vi "Energy Detection.vi"() -> ()   [LabVIEW 2012]
uses:
  <vilib>/measure/maspectr.llb/FFT Power Spectrum and PSD for 1 Chan.vi
  <instrlib>/niUSRP/niUSRP Fetch Rx Data (CDB Cluster).vi
  <vilib>/addons/Modulation/Digital/General/MT Generate PSK System Parameters(M).vi
  <instrlib>/niUSRP/niUSRP Write Tx Data (CDB Cluster).vi
  <vilib>/addons/Modulation/niDMT.lvlib
  <vilib>/measure/NI_MAPro.lvlib
panel:
  out "Power Spectrum / PSD":cluster{"f0":dbl, "df":dbl, "magnitude":dbl[]} {"magnitude" format="%.2p"; "f0" format="%0.2p"; "df" format="%0.2p"}
  out "SNR":dbl
  out "x/y":dbl
  in  "IQ rate 2":dbl=100000.0 format="%#_6p"
  in  "gain":dbl format="%#_6f"
  out "x+y 2":dbl
  out "CH1 is Free":bool
  out "CH2 is Free":bool
  out "CH3 is Free":bool
  out "CH4 is Free":bool
  out "String":string
  in  "millisecond multiple":u32
  out "millisecond timer value":u32
  out "Message Text 2":string
  out "Symbol Rate\n[symbols/sec]":dbl=25000.0 format="%#.6p"
  in  "BPSK System Parameters 9":T1={"Samples per Symbol"=8, "symbol map"=[], "Differential PSK"=enum."disable", "PSK type"=0} caption="BPSK System Parameters" {"PSK type" items=["normal", "shifted", "offset"]; "symbol map" format="%.3f"}
  in  "BPSK System Parameters 8":T1={"Samples per Symbol"=8, "symbol map"=[], "Differential PSK"=enum."disable", "PSK type"=0} caption="BPSK System Parameters" {"PSK type" items=["normal", "shifted", "offset"]; "symbol map" format="%.3f"}
  in  "BPSK System Parameters 7":T1={"Samples per Symbol"=8, "symbol map"=[], "Differential PSK"=enum."disable", "PSK type"=0} caption="BPSK System Parameters" {"PSK type" items=["normal", "shifted", "offset"]; "symbol map" format="%.3f"}
  in  "BPSK System Parameters 6":T1={"Samples per Symbol"=8, "symbol map"=[], "Differential PSK"=enum."disable", "PSK type"=0} caption="BPSK System Parameters" {"PSK type" items=["normal", "shifted", "offset"]; "symbol map" format="%.3f"}
  in  "BPSK System Parameters 5":T1={"Samples per Symbol"=8, "symbol map"=[], "Differential PSK"=enum."disable", "PSK type"=0} caption="BPSK System Parameters" {"PSK type" items=["normal", "shifted", "offset"]; "symbol map" format="%.3f"}
  in  "BPSK System Parameters 4":T1={"Samples per Symbol"=8, "symbol map"=[], "Differential PSK"=enum."disable", "PSK type"=0} caption="BPSK System Parameters" {"PSK type" items=["normal", "shifted", "offset"]; "symbol map" format="%.3f"}
  in  "BPSK System Parameters 3":T1={"Samples per Symbol"=8, "symbol map"=[], "Differential PSK"=enum."disable", "PSK type"=0} caption="BPSK System Parameters" {"PSK type" items=["normal", "shifted", "offset"]; "symbol map" format="%.3f"}
  in  "Tab Control":T2(tab)
  in  "Enter control signal (1,2 or 3)":string
  in  "Packet Parameters":T3={"Guard Bits "=30, "Sync Bits"=20, "Message Bits"=128}
  in  "Packet Pad \n[samples]":i32=200
  in  "Blank Frame \n[samples]":i32=500
  out "Number of Packets in Message":i32=46
  in  "PN sequence order\nfor Sync Bits":i32=31 caption="PN sequence order (9)"
  in  "Packet Repeat":i32=2
  in  "Pulse Shaping Filter Parameters":T4={"Alpha"=0.5, "Filter Length"=6, "TX Filter"=enum."Root Raised Cos"} caption="Pulse Shaping Filter" {"Alpha" format="%.2f"}
  in  "USRP IP address":refnum<k15>="192.168.10.2"
  out "error out":errorcluster
  in  "Queue Length":i32=10
  in  "stop":bool
  out "result":bool
  out "Constellation Graph":T5(graph)
  in  "autoscale":bool
  in  "millisecond multiple 2":u32
  out "millisecond timer value 2":u32
  out "x = y?":bool
  out "Boolean":bool
  out "M-PSK (4)":i32
  out "Enter control signal (1,2 or 3) 2":string
  out "Tx Frequency [Hz]":dbl
  out "x+y":dbl
  in  "Carrier Frequency":dbl
  in  "active antenna":string
  in  "IQ rate":dbl=100000.0 format="%#_6p"
  out "coerced carrier frequency":dbl=100000.0 format="%#_6p"
  out "coerced gain":dbl format="%#_6f"
  # "Guard\nBand"
  # "Sync\nSeq"
  # "Packet\nNumber"
  # "Pad\nData"
  # "Blank\nFrame"
  # "Data"
types:
  T1 = cluster{"Samples per Symbol":i32, "symbol map":cdb[], "Differential PSK":enum16{"disable", "enable"}, "PSK type":u16}
  T2 = enum32{"Specify Message", "Specify Packet", "Specify Modulation", "Tx Parameters", "Debug"}
  T3 = cluster{"Guard Bits ":i32, "Sync Bits":i32, "Message Bits":i32}
  T4 = cluster{"Alpha":dbl, "Filter Length":i32, "TX Filter":enum16{"none", "Raised Cosine", "Root Raised Cos", "Gaussian"}}
  T5 = cluster{"Decimated Array":dbl[], "Decimated Array":dbl[]}[]
  T6 = cluster{"samples per symbol (16)":i32, "symbol map":cdb[], "differential PSK":enum16{"disable", "enable"}, "PSK type":u16}
  T7 = cluster{"s? t:f":cluster{"t0":dbl, "dt":dbl, "Y":cdb[]}, i32}
  T8 = cluster{"output complex waveform":cluster{"t0":dbl, "dt":dbl, "Y":cdb[]}, i32}
  T9 = cluster{"constellation":dbl[], "oversampled data":dbl[]}[]
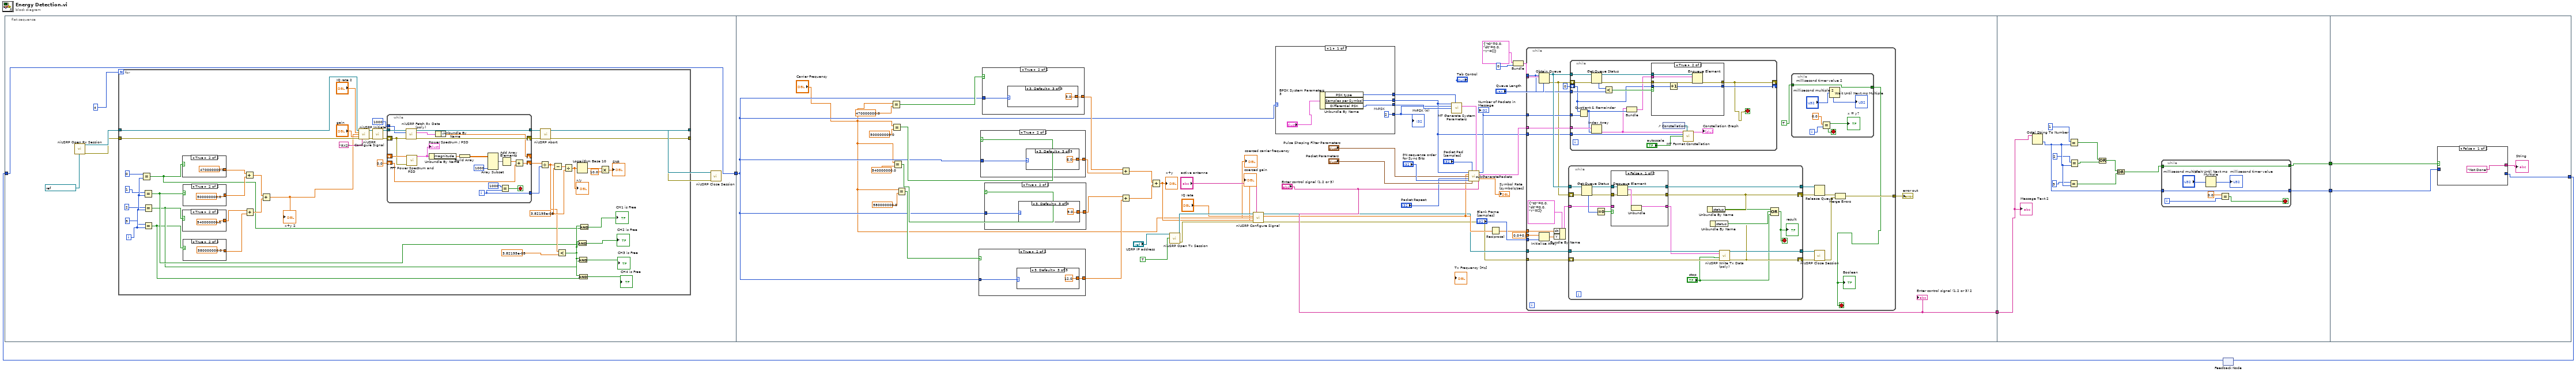
[diagram p0: block diagram]
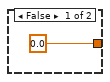
[diagram p2: hidden frame]
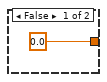
[diagram p3: hidden frame]
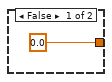
[diagram p4: hidden frame]
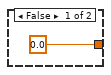
[diagram p5: hidden frame]
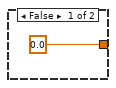
[diagram p6: hidden frame]
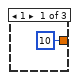
[diagram p7: hidden frame]
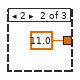
[diagram p8: hidden frame]
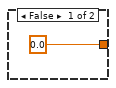
[diagram p9: hidden frame]
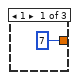
[diagram p10: hidden frame]
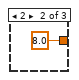
[diagram p11: hidden frame]
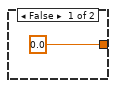
[diagram p12: hidden frame]
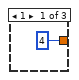
[diagram p13: hidden frame]
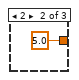
[diagram p14: hidden frame]
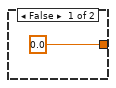
[diagram p15: hidden frame]
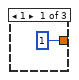
[diagram p16: hidden frame]
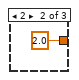
[diagram p17: hidden frame]
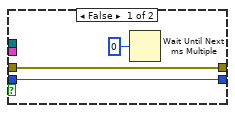
[diagram p18: hidden frame]
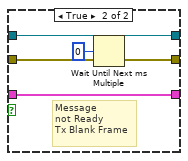
[diagram p19: hidden frame]
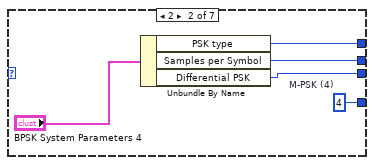
[diagram p20: hidden frame]
diagram:
  n1 = flat-sequence {
    tunnel: w1 -> [w13]
    tunnel: [w13] -> w2
    tunnel: ["Enter control signal (1,2 or 3)"] -> w6
    tunnel: w2 -> [w94]
    tunnel: w6 -> [w283]
    tunnel: [w285] -> w5
    tunnel: [w284] -> w4
    tunnel: w5 -> [w304]
    tunnel: w4 -> [w303]
    tunnel: [w302] -> w3
    frame #0 {
      n2 = call <instrlib>:"niUSRP Open Rx Session.vi"("device names"=refnum<k15> "192.168.10.4") -> ("session handle out"=w12:refnum<k15>, "error out"=w11:errorcluster)  [unwired: 13 in]
      n3 = for {
        N: 4 -> [_]
        tunnel: w12 -> [w59]
        tunnel: w11 -> [w56]
        tunnel: [w42] -> w8
        tunnel: [w41] -> w7
        i -> [w36]
        w38 = 3.82195e-05 ("y")
        n4 = Equal?(x=0, y=w36) -> (x = y?=w21:bool)
        n5 = Equal?(x=1, y=w36) -> (x = y?=w20:bool)
        n6 = Equal?(x=2, y=w36) -> (x = y?=w19:bool)
        n7 = Equal?(x=3, y=w36) -> (x = y?=w18:bool)
        n8 = case shown="True" w21 {
          tunnel: [0.0 470000000.0] -> w31
          frame False {
          }
          frame True {
          }
        }
        n9 = case shown="True" w19 {
          tunnel: [0.0 540000000.0] -> w29
          frame False {
          }
          frame True {
          }
        }
        n10 = case shown="True" w20 {
          tunnel: [0.0 500000000.0] -> w30
          frame False {
          }
          frame True {
          }
        }
        n11 = case shown="True" w18 {
          tunnel: [0.0 580000000.0] -> w26
          frame False {
          }
          frame True {
          }
        }
        n12 = Add(x=w31, y=w30) -> (x+y=w28:dbl)
        n13 = Add(x=w29, y=w26) -> (x+y=w27:dbl)
        n14 = Add(x=w28, y=w27) -> (x+y=w23:dbl)
        "x+y 2" <- w23
        n15 = call <instrlib>:"niUSRP Configure Signal.vi"("session handle"=w59, "IQ rate"="IQ rate 2", "carrier frequency"=w23, "gain"="gain", "error in (no error)"=w56, "active antenna"="RX2") -> ("session handle out"=w58:refnum<k15>, "error out"=w57:errorcluster)  [unwired: 5 in, 3 out]
        n16 = call <instrlib>:"niUSRP Initiate.vi"("session handle"=w58, "error in (no error)"=w57) -> ("session handle out"=w55:refnum<k15>, "error out"=w54:errorcluster)  [unwired: 12 in]
        n17 = while {
          tunnel: w55 -> [w86]
          shift-right: [w70] -> w53
          shift-left: w54 -> [w83]
          tunnel: [w85] -> w52
          shift-right: [w68] -> _
          shift-left: _ -> [w84]
          shift-right: [w77] -> w50
          shift-left: 0.0 -> [w78]
          tunnel: [w72] -> w49
          tunnel: 1000 -> [w75]
          i -> [w72]
          stop <- w71 stop-if-true
          n18 = call-poly <instrlib>:"niUSRP Fetch Rx Data (poly).vi"("session handle"=w86, "number of samples"=w75, "error in (no error)"=w83) -> ("session handle out"=w85:refnum<k15>, "data"=w69:cluster{"t0":dbl, "dt":dbl, "Y":cdb[]}, "error out"=w70:errorcluster)  [unwired: 9 in, 1 out]
          n19 = call-poly <vilib>:"FFT Power Spectrum and PSD.vi"("error in (no error)"=w83, "time signal"=w84) -> ("Power Spectrum / PSD"=w82:cluster{"f0":dbl, "df":dbl, "magnitude":dbl[]})  [unwired: 6 in, 3 out]
          "Power Spectrum / PSD" <- w82
          n20 = Unbundle By Name(w82) -> ("magnitude"=w81:dbl[])
          n21 = Unbundle By Name(w69) -> ("Y"=w68:cdb[])
          n22 = Build Array(w81) -> (w80:dbl[][])
          n23 = Array Subset(array=w80, length (col)=1000 ("length")) -> (w79:dbl[][])  [unwired: 3 in]
          n24 = Equal?(x=1000, y=w72) -> (x = y?=w71:bool)
          n25 = Add Array Elements(numeric array=w79) -> (sum=w76:dbl)
          n26 = Add(x=w76, y=w78) -> (x+y=w77:dbl)
        }
        n27 = Divide(x=w50, y=w49) -> (x/y=w25:dbl)
        n28 = call <instrlib>:"niUSRP Abort.vi"("session handle"=w52, "error in (no error)"=w53) -> ("session handle out"=w42:refnum<k15>, "error out"=w41:errorcluster)  [unwired: 12 in]
        n29 = Subtract(x=w25, y=w38) -> (x-y=w37:dbl)
        n30 = Less?(x=w25, y=3.82195e-05) -> (x < y?=w22:bool)
        n31 = Divide(x=w37, y=w38) -> (x/y=w48:dbl)
        "x/y" <- w48
        n32 = Logarithm Base 10(1:w48) -> (0:w47:dbl)
        n33 = And(x=w22, y=w20) -> (x .and. y?=→"CH2 is Free":bool)
        n34 = And(x=w22, y=w19) -> (x .and. y?=→"CH3 is Free":bool)
        n35 = And(x=w22, y=w18) -> (x .and. y?=→"CH4 is Free":bool)
        n36 = And(x=w22, y=w21) -> (x .and. y?=→"CH1 is Free":bool)
        n37 = Multiply(x=w47, y=10.0) -> (x*y=→"SNR":dbl)
      }
      n38 = call <instrlib>:"niUSRP Close Session.vi"("session handle"=w8, "error in (no error)"=w7) -> ()  [unwired: 13 in, 1 out]
    }
    frame #1 {
      n39 = Equal?(x="Carrier Frequency", y=470000000.0) -> (x = y?=w95:bool)
      n40 = Equal?(x="Carrier Frequency", y=500000000.0) -> (x = y?=w96:bool)
      n41 = Equal?(x="Carrier Frequency", y=540000000.0) -> (x = y?=w97:bool)
      n42 = Equal?(x="Carrier Frequency", y=580000000.0) -> (x = y?=w98:bool)
      n43 = case shown="True" w98 {
        tunnel: [0.0 w138] -> w103
        tunnel: w94 -> [_ w139]
        frame False {
        }
        frame True {
          n44 = case shown="3, Default" w139 {
            tunnel: [10 11.0 12.0] -> w138
            frame 1 {
            }
            frame 2 {
            }
            frame 3, Default {
            }
          }
        }
      }
      n45 = case shown="True" w96 {
        tunnel: [0.0 w150] -> w105
        tunnel: w94 -> [_ w151]
        frame False {
        }
        frame True {
          n46 = case shown="3, Default" w151 {
            tunnel: [4 5.0 6.0] -> w150
            frame 1 {
            }
            frame 2 {
            }
            frame 3, Default {
            }
          }
        }
      }
      n47 = case shown="True" w95 {
        tunnel: [0.0 w156] -> w106
        tunnel: w94 -> [_ w157]
        frame False {
        }
        frame True {
          n48 = case shown="3, Default" w157 {
            tunnel: [1 2.0 3.0] -> w156
            frame 1 {
            }
            frame 2 {
            }
            frame 3, Default {
            }
          }
        }
      }
      n49 = case shown="True" w97 {
        tunnel: [0.0 w144] -> w104
        tunnel: w94 -> [_ w145]
        frame False {
        }
        frame True {
          n50 = case shown="3, Default" w145 {
            tunnel: [7 8.0 9.0] -> w144
            frame 1 {
            }
            frame 2 {
            }
            frame 3, Default {
            }
          }
        }
      }
      n51 = Add(x=w106, y=w105) -> (x+y=w108:dbl)
      n52 = Add(x=w104, y=w103) -> (x+y=w107:dbl)
      n53 = Add(x=w108, y=w107) -> (x+y=w93:dbl)
      "x+y" <- w93
      n54 = call <instrlib>:"niUSRP Open Tx Session.vi"("device names"="USRP IP address", "reset"=TRUE) -> ("session handle out"=w111:refnum<k15>, "error out"=w112:errorcluster)  [unwired: 12 in]
      n55 = call <instrlib>:"niUSRP Configure Signal.vi"("session handle"=w111, "IQ rate"="IQ rate", "carrier frequency"="Carrier Frequency", "gain"=w93, "error in (no error)"=w112, "active antenna"="active antenna") -> ("session handle out"=w110:refnum<k15>, "coerced IQ rate"=w113:dbl, "coerced carrier frequency"=→"coerced carrier frequency":dbl, "coerced gain"=→"coerced gain":dbl, "error out"=w109:errorcluster)  [unwired: 5 in]
      n56 = case shown="1" w94 {
        tunnel: [w249 w254 w261 w266 w271 w277 w280] -> w117
        tunnel: [w250 w255 w260 w265 w270 w276 w281] -> w136
        tunnel: [w252 w257 w262 w267 w269 w275 0 ("M-PSK (4)")] -> w128
        tunnel: [w251 w256 w259 w264 w272 w274 w282] -> w122
        frame 1 {
          w252 = 2  # M-PSK
          n57 = Unbundle By Name("BPSK System Parameters 3") -> ("PSK type"=w251:u16, "Samples per Symbol"=w249:i32, "Differential PSK"=w250:enum16{"disable", "enable"})
        }
        frame 2 {
          w257 = 4  # M-PSK (4)
          n58 = Unbundle By Name("BPSK System Parameters 4") -> ("PSK type"=w256:u16, "Samples per Symbol"=w254:i32, "Differential PSK"=w255:enum16{"disable", "enable"})
        }
        frame 4 {
          w262 = 4  # M-PSK (4)
          n59 = Unbundle By Name("BPSK System Parameters 5") -> ("PSK type"=w259:u16, "Samples per Symbol"=w261:i32, "Differential PSK"=w260:enum16{"disable", "enable"})
        }
        frame 5 {
          w267 = 4  # M-PSK (4)
          n60 = Unbundle By Name("BPSK System Parameters 6") -> ("PSK type"=w264:u16, "Samples per Symbol"=w266:i32, "Differential PSK"=w265:enum16{"disable", "enable"})
        }
        frame 3, Default {
          w269 = 8  # M-PSK (4)
          n61 = Unbundle By Name("BPSK System Parameters 7") -> ("PSK type"=w272:u16, "Samples per Symbol"=w271:i32, "Differential PSK"=w270:enum16{"disable", "enable"})
        }
        frame 6 {
          w275 = 16  # M-PSK (4)
          n62 = Unbundle By Name("BPSK System Parameters 8") -> ("PSK type"=w274:u16, "Samples per Symbol"=w277:i32, "Differential PSK"=w276:enum16{"disable", "enable"})
        }
        frame 7 {
          n63 = Unbundle By Name("BPSK System Parameters 9") -> ("PSK type"=w282:u16, "Samples per Symbol"=w280:i32, "Differential PSK"=w281:enum16{"disable", "enable"})
        }
      }
      "M-PSK (4)" <- w128
      n64 = call-poly <vilib>:"MT Generate System Parameters.vi"("samples per symbol (16)"=w117, "PSK type"=w122, "M-PSK (4)"=w128, "differential PSK"=w136) -> ("PSK system parameters"=w123:T6)  [unwired: 9 in, 2 out]
      n65 = call "subGeneratePackets.vi"("Samples per Symbol"=w117, "Packet Pad \n[samples]"="Packet Pad \n[samples]", "PSK system parameters"=w123, "Tx IQ Sampling\nRate [s/sec]"=w113, "Pulse Shaping Filter Parameters"="Pulse Shaping Filter Parameters", "Packet Repeat"="Packet Repeat", "PN sequence order\nfor Sync Bits"="PN sequence order\nfor Sync Bits", "Packet Parameters"="Packet Parameters", "Message Text"="Enter control signal (1,2 or 3)") -> ("Number of Packets"=w127:i32, "Packets"=w130:cluster{"t0":dbl, "dt":dbl, "Y":cdb[]}[], "Symbol Rate"=→"Symbol Rate\n[symbols/sec]":dbl)  [unwired: 4 in]
      "Number of Packets in Message" <- w127
      n66 = Reciprocal(x=w113) -> (1/x=w129:dbl)
      n67 = Bundle("s? t:f"=cluster{"t0":dbl, "dt":dbl, "Y":cdb[]} {"t0"=0.0, "dt"=0.0, "Y"=[]}, 0) -> (w132:T7)  [unwired: 1 in]
      n68 = while {
        tunnel: cdb 0.0+0.0i ("element") -> [w185]
        tunnel: "Blank Frame \n[samples]" -> [w184]
        tunnel: w132 -> [w178]
        tunnel: "Queue Length" -> [w176]
        tunnel: w130 -> [w175]
        tunnel: w109 -> [w174]
        tunnel: w129 -> [w171]
        tunnel: w110 -> [w170]
        tunnel: w127 -> [w169]
        tunnel: [w164] -> w121
        tunnel: w117 -> [w163]
        stop <- w161 stop-if-true
        n69 = Obtain Queue(max queue size (-1, unlimited)=w176, element data type=w178) -> (queue out=w183:refnum<queue>, error out=w167:errorcluster)  [unwired: 3 in, 1 out]
        n70 = Initialize Array(w185, w184) -> (w182:cdb[])
        n71 = Bundle By Name(cluster=cluster{"t0":dbl, "dt":dbl, "Y":cdb[]} {"t0"=0.0, "dt"=0.0, "Y"=[]} ("s? t:f"), "dt"=w171, "Y"=w182) -> (w181:cluster{"t0":dbl, "dt":dbl, "Y":cdb[]})
        n72 = while {
          tunnel: w170 -> [w228]
          shift-right: [w225] -> w173
          shift-left: w174 -> [w229]
          tunnel: w183 -> [w237]
          tunnel: w181 -> [w234]
          tunnel: [w233] -> w180
          tunnel: [w227] -> w172
          shift-right: [w223] -> w179
          shift-left: w167 -> [w230]
          stop <- w220 stop-if-true
          n73 = Get Queue Status(queue=w237, error in (no error)=w230) -> (queue out=w232:refnum<queue>, error out=w231:errorcluster, # elements in queue=w236:i32)  [unwired: 1 in, 5 out]
          n74 = Equal To 0?(x=w236) -> (x = 0?=w235:bool)
          n75 = case shown="False" w235 {
            tunnel: w234 -> [_ w247]
            tunnel: [w239 w247] -> w221
            tunnel: [w243 w245] -> w233
            tunnel: [w238 w246] -> w223
            tunnel: w232 -> [w242 w245]
            tunnel: w231 -> [w241 w246]
            frame False {
              n76 = Dequeue Element(queue=w242, error in (no error)=w241) -> (queue out=w243:refnum<queue>, element=w240:T7, error out=w238:errorcluster)  [unwired: 1 in, 1 out]
              n77 = Unbundle(w240) -> ("s? t:f"=w239:cluster{"t0":dbl, "dt":dbl, "Y":cdb[]})  [unwired: 1 out]
            }
            frame True {
              # "Message\nnot Ready\nTx Blank Frame"
              n78 = Wait Until Next ms Multiple(millisecond multiple=u32 0) -> ()  [unwired: 1 out]
            }
          }
          n79 = Unbundle By Name(w223) -> ("status"=w222:bool)
          n80 = call-poly <instrlib>:"niUSRP Write Tx Data (poly).vi"("session handle"=w228, "data"=w221, "end of data?"="stop", "error in (no error)"=w229) -> ("session handle out"=w227:refnum<k15>, "error out"=w225:errorcluster)  [unwired: 10 in]
          n81 = Unbundle By Name(w225) -> ("status"=w226:bool)
          n82 = Compound Arithmetic op=OR(w222, w226, "stop") -> (w220:bool)
          "result" <- w220
        }
        n83 = while {
          tunnel: w183 -> [w210]
          shift-right: [w203] -> _
          shift-left: 0 -> [w199]
          tunnel: w175 -> [w200]
          tunnel: w176 -> [w202]
          tunnel: w169 -> [w201]
          shift-right: [w192] -> _
          shift-left: w167 -> [w205]
          tunnel: w163 -> [w195]
          stop <- w192 stop-if-true
          n84 = Quotient & Remainder(x=w199, y=w201) -> (x-y*floor(x/y)=w198:i32)  [unwired: 1 out]
          n85 = Index Array(array=w200, index=w198) -> (element=w193:cluster{"t0":dbl, "dt":dbl, "Y":cdb[]})
          n86 = Get Queue Status(queue=w210, error in (no error)=w205) -> (queue out=w209:refnum<queue>, error out=w206:errorcluster, # elements in queue=w208:i32)  [unwired: 1 in, 5 out]
          n87 = Less?(x=w208, y=w202) -> (x < y?=w207:bool)
          n88 = Bundle("output complex waveform"=w193, w198) -> (w204:T8)  [unwired: 1 in]
          n89 = case shown="True" w207 {
            tunnel: w206 -> [w211 w219]
            tunnel: w209 -> [_ w218]
            tunnel: [w211 w217] -> w192
            tunnel: w204 -> [_ w216]
            tunnel: w199 -> [w213 w215]
            tunnel: [w213 w214] -> w203
            frame False {
              n90 = Wait Until Next ms Multiple(millisecond multiple=u32 0) -> ()  [unwired: 1 out]
            }
            frame True {
              n91 = Increment(x=w215) -> (x+1=w214:i32)
              n92 = Enqueue Element(queue=w218, element=w216, error in (no error)=w219) -> (error out=w217:errorcluster)  [unwired: 1 in, 2 out]
            }
          }
          n93 = control-ref of="Constellation Graph"() -> (w196:refnum<vi>)
          n94 = call <vilib>:"MT Format Constellation.vi"("waveform"=w193, "constellation reference"=w196, "samples per symbol"=w195, "autoscale"="autoscale") -> ("constellation graph"=→"Constellation Graph":T9)  [unwired: 1 in, 10 out]
        }
        n95 = while {
          tunnel: TRUE -> [w191]
          tunnel: [w191] -> w161
          i -> [w189]
          stop <- w188 stop-if-true
          n96 = Equal?(x=0.0, y=w189) -> (x = y?=w188:bool)
          "x = y?" <- w188
          n97 = Wait Until Next ms Multiple(millisecond multiple="millisecond multiple 2") -> (millisecond timer value=→"millisecond timer value 2":u32)
        }
        "Boolean" <- w161
        n98 = Release Queue(queue=w180, error in (no error)=w179) -> (error out=w166:errorcluster)  [unwired: 3 out]
        n99 = call <instrlib>:"niUSRP Close Session.vi"("session handle"=w172, "error in (no error)"=w173) -> ("error out"=w165:errorcluster)  [unwired: 13 in]
        n100 = Merge Errors(w166, w165) -> (w164:errorcluster)
      }
      "error out" <- w121
      "Enter control signal (1,2 or 3) 2" <- "Enter control signal (1,2 or 3)"
    }
    frame #2 {
      n101 = Octal String To Number(4:w283) -> (0:w289:u32)  [unwired: 2 in, 1 out]
      n102 = Equal?(x=3, y=w289) -> (x = y?=w291:bool)
      n103 = Equal?(x=1, y=w289) -> (x = y?=w294:bool)
      n104 = Equal?(x=2, y=w289) -> (x = y?=w293:bool)
      n105 = Or(x=w294, y=w293) -> (x .or. y?=w292:bool)
      n106 = Or(x=w292, y=w291) -> (x .or. y?=w290:bool)
      n107 = while {
        tunnel: w290 -> [w299]
        tunnel: [w299] -> w285
        tunnel: w289 -> [w298]
        tunnel: [w298] -> w284
        i -> [w296]
        stop <- w295 stop-if-true
        n108 = Wait Until Next ms Multiple(millisecond multiple="millisecond multiple") -> (millisecond timer value=→"millisecond timer value":u32)
        n109 = Equal?(x=0.0, y=w296) -> (x = y?=w295:bool)
      }
      "Message Text 2" <- w283
    }
    frame #3 {
      n110 = case shown="False" w304 {
        tunnel: ["Not Done" "Switching Done"] -> w305
        tunnel: [_ w307] -> w302
        tunnel: w303 -> [_ w307]
        frame False {
        }
        frame True {
        }
      }
      "String" <- w305
    }
  }
  n111 = feedback #1() -> (w1:u32)  [unwired: 1 in]
  n112 = feedback-in #1(w3) -> ()
